vi "1C SmallRCSensorConsole.vi"() -> ()   [LabVIEW 2011]
uses:
  2-RIO/2 Typedefs/Velocity.ctl
  2-RIO/2 Typedefs/Boat Orientation.ctl
  2-RIO/2 Typedefs/Boat Position.ctl
  2-RIO/2 Typedefs/Velocity as Direction and Speed.ctl
panel:
  out "Absolute Wind":T1
  in  "Add Randomness\nTo Wind Measurement":bool
  out "Apparent Wind":T1
  in  "Wind Manual\nInput":T2 {"Direction" scale=0.0..6.283}
  out "Actual\nWind Velocity":T1
  out "Boat Velocity":T1
  out "Boat Position":T3
  out "Boat Orientation":T4 scale=0.0..6.283
  out "Overhead Image":T5(plugin-control)
  # "UNFINISHED\nTODO: finish camera interpreter and test!"
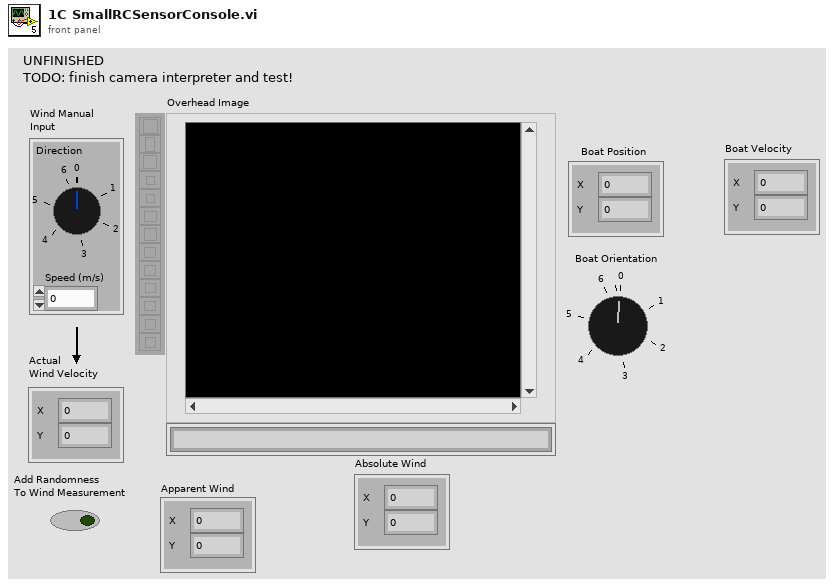
[diagram p1: front panel]
types:
  T1 = typedef "Velocity.ctl" = cluster{"X":dbl, "Y":dbl}
  T2 = typedef "Velocity as Direction and Speed.ctl" = cluster{"Speed (m/s)":dbl, "Direction":dbl}
  T3 = typedef "Boat Position.ctl" = cluster{"X":dbl, "Y":dbl}
  T4 = typedef "Boat Orientation.ctl" = dbl
  T5 = typedef "IMAQ Image.ctl" = refnum<image>
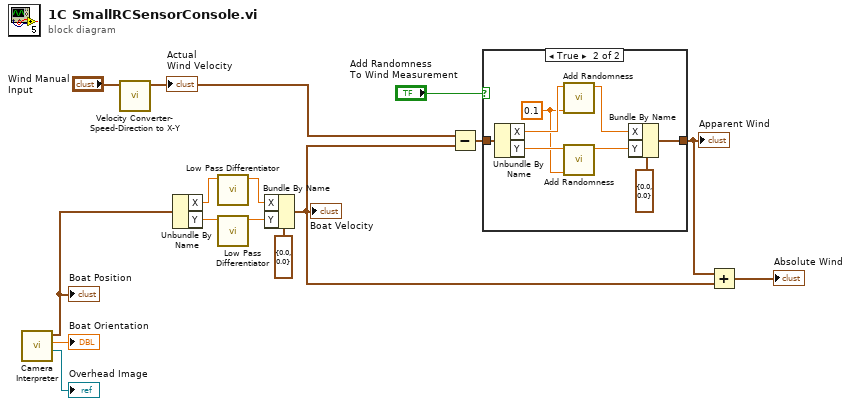
[diagram p0: block diagram]
diagram:
  n1 = call "Camera Interpreter.vi"() -> ("Overhead Image"=→"Overhead Image":T5, "Boat Orientation"=→"Boat Orientation":T4, "Boat Position"=w13:T3)  [unwired: 9 in]
  "Boat Position" <- w13
  n2 = call "Velocity Converter- Speed-Direction to X-Y.vi"("Velocity as\nDirection/Speed"="Wind Manual\nInput") -> ("Velocity as X/Y"=w6:T1)  [unwired: 10 in]
  "Actual\nWind Velocity" <- w6
  n3 = Unbundle By Name(w13) -> ("X"=w12:dbl, "Y"=w11:dbl)
  n4 = call "Low Pass Differentiator.vi"("X"=w12) -> ("dX, smoothed"=w8:dbl)  [unwired: 10 in]
  n5 = call "Low Pass Differentiator.vi"("X"=w11) -> ("dX, smoothed"=w9:dbl)  [unwired: 10 in]
  n6 = Bundle By Name(cluster=T1 {"X"=0.0, "Y"=0.0} ("Boat Velocity 2"), "X"=w8, "Y"=w9) -> (w2:T1)
  "Boat Velocity" <- w2
  n7 = Subtract(x=w6, y=w2) -> (x-y=w5:T1)
  n8 = case shown="True" "Add Randomness\nTo Wind Measurement" {
    tunnel: [w16 w24] -> w3
    tunnel: w5 -> [w16 w22]
    frame False {
    }
    frame True {
      w17 = 0.1 ("Amplitude\n(default 1)")
      n9 = Unbundle By Name(w22) -> ("X"=w21:dbl, "Y"=w20:dbl)
      n10 = call "Add Randomness.vi"("Amplitude\n(default 1)"=w17, "Numeric in"=w21) -> ("Numeric out"=w18:dbl)  [unwired: 9 in]
      n11 = call "Add Randomness.vi"("Amplitude\n(default 1)"=w17, "Numeric in"=w20) -> ("Numeric out"=w19:dbl)  [unwired: 9 in]
      n12 = Bundle By Name(cluster=T1 {"X"=0.0, "Y"=0.0} ("Boat Velocity 2"), "X"=w18, "Y"=w19) -> (w24:T1)
    }
  }
  "Apparent Wind" <- w3
  n13 = Add(x=w3, y=w2) -> (x+y=→"Absolute Wind":T1)
